vi "FramePack.vi"(3 "error in":errorcluster caption="错误输入（无错误）", 4 "F0?":bool, 5 "SNorDevID":cluster{"SN":string, "DevID":string}, 6 "FramePara":T1) -> (0 "error out":errorcluster caption="错误输出", 1 "连接的字符串":string, 2 "CMD":string)   [LabVIEW 2013]
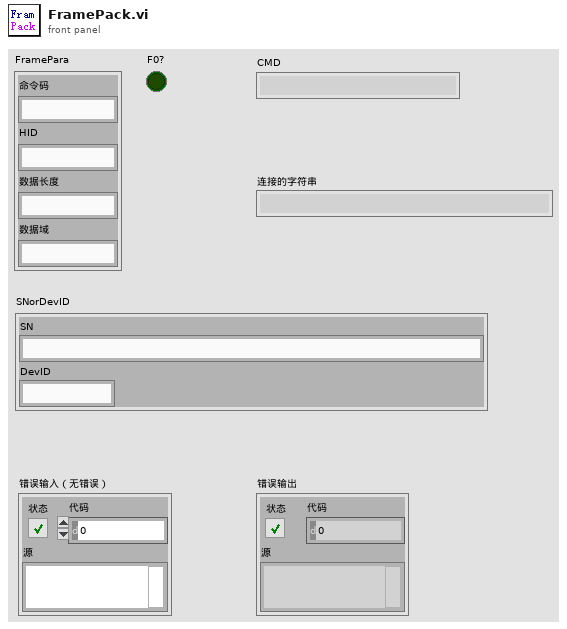
[diagram p1: front panel]
types:
  T1 = cluster{"命令码":string, "HID":string, "数据长度":string, "数据域":string}
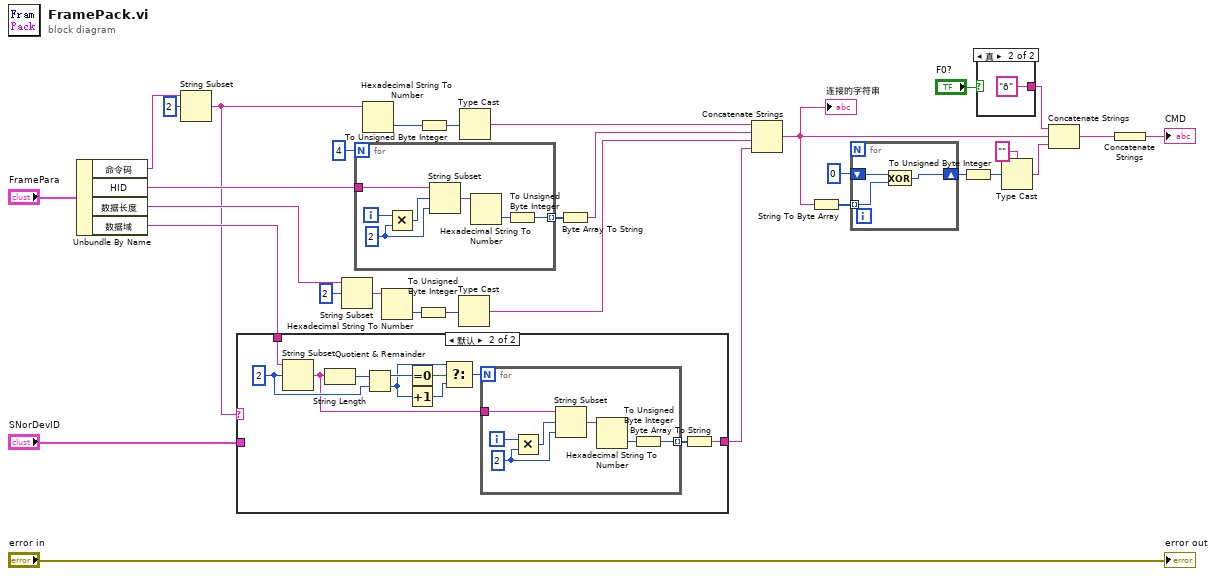
[diagram p0: block diagram]
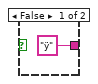
[diagram p2: hidden frame]
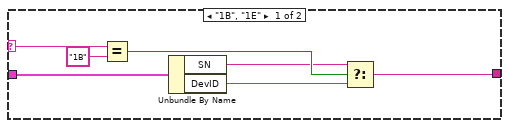
[diagram p3: hidden frame]
diagram:
  n1 = Unbundle By Name("FramePara") -> ("命令码"=w28:string, "HID"=w25:string, "数据长度"=w20:string, "数据域"=w19:string)
  n2 = String Subset(string=w28, offset (0)=2 ("偏移量(0)")) -> (substring=w3:string)  [unwired: 1 in]
  n3 = case shown="默认" w3 {
    selector: w3 -> [w39 _]
    tunnel: w19 -> [_ w50]
    tunnel: [w34 w49] -> w16
    tunnel: "SNorDevID" -> [w36 _]
    frame "1B", "1E" {
      n4 = Equal?(x=w39, y="1B") -> (x = y?=w37:bool)
      n5 = Unbundle By Name(w36) -> ("SN"=w35:string, "DevID"=w33:string)
      n6 = Select(t=w35, s=w37, f=w33) -> (s? t:f=w34:string)
    }
    frame Default {
      w47 = 2 ("偏移量(0)")
      n7 = String Subset(string=w50, offset (0)=w47) -> (substring=w40:string)  [unwired: 1 in]
      n8 = String Length(string=w40) -> (length=w48:i32)
      n9 = Quotient & Remainder(x=w48, y=w47) -> (x-y*floor(x/y)=w46:i32, floor(x/y)=w43:i32)
      n10 = Equal To 0?(x=w46) -> (x = 0?=w45:bool)
      n11 = Increment(x=w43) -> (x+1=w44:i32)
      n12 = Select(t=w43, s=w45, f=w44) -> (s? t:f=w41:i32)
      n13 = for {
        N: w41 -> [_]
        tunnel: w40 -> [w55]
        tunnel: [w51] -> w42 mode=indexing
        i -> [w57]
        w54 = 2
        n14 = Multiply(x=w57, y=w54) -> (x*y=w56:i32)
        n15 = String Subset(string=w55, offset (0)=w56, length (rest)=w54) -> (substring=w53:string)
        n16 = Hexadecimal String To Number(string=w53) -> (number=w52:u32)  [unwired: 2 in, 1 out]
        n17 = To Unsigned Byte Integer(number=w52) -> (unsigned 8bit integer=w51:u8)
      }
      n18 = Byte Array To String(unsigned byte array=w42) -> (string=w49:string)
    }
  }
  n19 = String Subset(string=w20, offset (0)=2 ("偏移量(0)")) -> (substring=w23:string)  [unwired: 1 in]
  n20 = for {
    N: 4 -> [_]
    tunnel: w25 -> [w62]
    tunnel: [w58] -> w26 mode=indexing
    i -> [w64]
    w61 = 2
    n21 = Multiply(x=w64, y=w61) -> (x*y=w63:i32)
    n22 = String Subset(string=w62, offset (0)=w63, length (rest)=w61) -> (substring=w60:string)
    n23 = Hexadecimal String To Number(string=w60) -> (number=w59:u32)  [unwired: 2 in, 1 out]
    n24 = To Unsigned Byte Integer(number=w59) -> (unsigned 8bit integer=w58:u8)
  }
  n25 = Hexadecimal String To Number(string=w3) -> (number=w30:u32)  [unwired: 2 in, 1 out]
  n26 = Hexadecimal String To Number(string=w23) -> (number=w22:u32)  [unwired: 2 in, 1 out]
  n27 = To Unsigned Byte Integer(number=w22) -> (unsigned 8bit integer=w21:u8)
  n28 = To Unsigned Byte Integer(number=w30) -> (unsigned 8bit integer=w31:u8)
  n29 = Type Cast(x=w21) -> (*(type *) &x=w4:string)  [unwired: 1 in]
  n30 = Type Cast(x=w31) -> (*(type *) &x=w18:string)  [unwired: 1 in]
  n31 = Byte Array To String(unsigned byte array=w26) -> (string=w17:string)
  n32 = Concatenate Strings(w18, w17, w4, w16) -> (w10:string)
  "连接的字符串" <- w10
  n33 = String To Byte Array(string=w10) -> (unsigned byte array=w14:u8[])
  n34 = for {
    shift-right: [w65] -> w13
    shift-left: u8 0 -> [w67]
    tunnel: w14 -> [w66] mode=indexing
    n35 = Exclusive Or(1:w66, 2:w67) -> (0:w65:u8)
  }
  n36 = To Unsigned Byte Integer(number=w13) -> (unsigned 8bit integer=w12:u8)
  n37 = case shown="真" "F0?" {
    tunnel: ["ÿ" "ð"] -> w8
    frame False {
    }
    frame True {
    }
  }
  n38 = Type Cast(type="", x=w12) -> (*(type *) &x=w11:string)
  n39 = Concatenate Strings(w8, w10, w11) -> (w7:string)
  n40 = Concatenate Strings(w7) -> (→"CMD":string)
  "error out" <- "error in"
